vi "Get Priority Target.vi"(11 "Target Info":T1(array[cluster])) -> (3 "Cluster":T2)   [LabVIEW 2011]
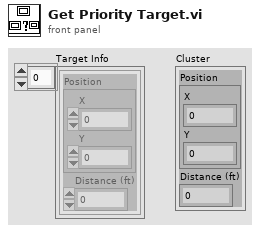
[diagram p1: front panel]
types:
  T1 = cluster{"Position":cluster{"X":dbl, "Y":dbl}, "Distance (ft)":dbl}[]
  T2 = cluster{"Position":cluster{"X":dbl, "Y":dbl}, "Distance (ft)":dbl}
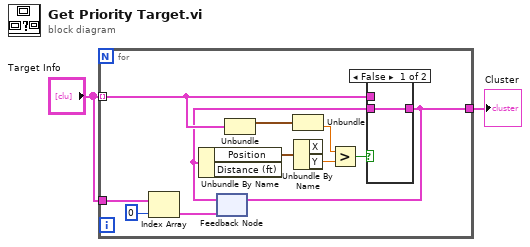
[diagram p0: block diagram]
diagram:
  n1 = for {
    tunnel: "Target Info" -> [w10] mode=indexing
    tunnel: [w6] -> w2
    tunnel: "Target Info" -> [w5]
    n2 = Index Array(array=w5, index=0) -> (element=w3:T2)
    n3 = feedback #1(w3) -> (w8:T2)
    n4 = Unbundle By Name(w8) -> ("Position"=w9:cluster{"X":dbl, "Y":dbl})  [unwired: 1 out]
    n5 = Unbundle(w10) -> ("Position"=w13:cluster{"X":dbl, "Y":dbl})  [unwired: 1 out]
    n6 = Unbundle(w13) -> ("Y"=w11:dbl)  [unwired: 1 out]
    n7 = Unbundle By Name(w9) -> ("Y"=w7:dbl)  [unwired: 1 out]
    n8 = Greater?(x=w11, y=w7) -> (0:w12:bool)
    n9 = case shown="False" w12 {
      tunnel: [w14 w15] -> w6
      tunnel: w10 -> [_ w15]
      tunnel: w8 -> [w14 _]
      frame False {
      }
      frame True {
      }
    }
    n10 = feedback-in #1(w6) -> ()
  }
  "Cluster" <- w2
